vi "Write Name.vi"(8 "error in (no error)":errorcluster, 10 "Name":string, 11 "Paquetes Disponibles in":refnum<class "Paquetes Disponibles.lvclass">) -> (0 "error out":errorcluster, 3 "Paquetes Disponibles out":refnum<class "Paquetes Disponibles.lvclass">)   [LabVIEW 2020, in "Paquetes Disponibles.lvlib" / "Paquetes Disponibles.lvclass"]
uses:
  Paquetes Disponibles.lvclass
  Paquetes Disponibles.lvclass/Paquetes Disponibles.ctl
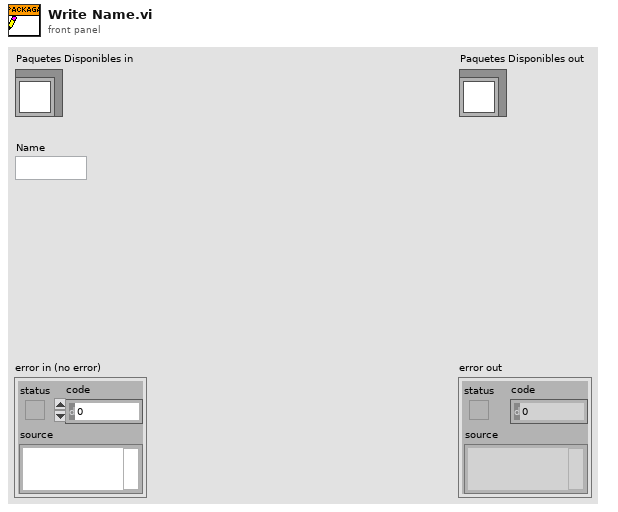
[diagram p1: front panel]
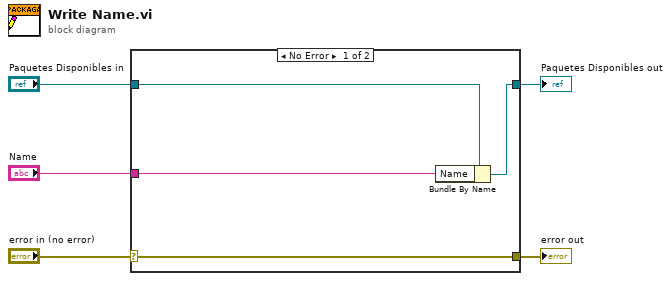
[diagram p0: block diagram]
diagram:
  n1 = case shown="No Error" "error in (no error)" {
    selector: "error in (no error)" -> [w9 w10]
    tunnel: [w9 w10] -> w4
    tunnel: [w7 w11] -> w2
    tunnel: "Paquetes Disponibles in" -> [w8 w11]
    tunnel: "Name" -> [w6 _]
    frame No Error {
      n2 = Bundle By Name(cluster=w8, "Name"=w6) -> (w7:refnum<class "Paquetes Disponibles.lvclass">)
    }
    frame Error {
    }
  }
  "error out" <- w4
  "Paquetes Disponibles out" <- w2
